vi "EnableDisableBankB - Right Click.vi"(8 "error in (no error)":errorcluster, 11 "Node Ptr":u64 format="%.0x") -> (0 "error out":errorcluster)   [LabVIEW 2015, in "DCM System Explorer.lvlib"]
uses:
  DCM System Explorer.lvlib
  System.Windows.Forms
  Shared/DCM Constants and GUIDs.vi
  Shared/DCM Properties.vi
  <vilib>/NI Veristand/Custom Device API/Set Item Property (Boolean).vi
  <vilib>/NI VeriStand/Custom Device API/Custom Device API.lvlib
  DCM Shared.lvlib
  <vilib>/NI Veristand/Custom Device Tools/Custom Device Utility Library/Custom Device Utility Library.lvlib
panel:
  in  "Tag":string
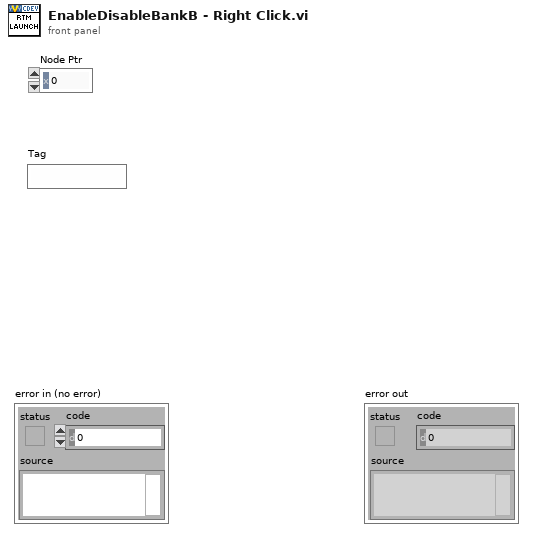
[diagram p1: front panel]
types:
  T1 = typedef "Custom Device API.lvlib/Custom Device Item Ref.ctl" = u64
  T2 = typedef "DCM - RT - DI.lvlib/Command.ctl" = cluster{"Mode":T3, "Digital Input":T4, "Default Phase Index":u8, "Frequency [Hz]":sgl, "Duration [s]":sgl, "Sweep [s]":sgl, "Injections":u16, "Command Sequence":T5[], "TDC Offset [CAD]":sgl, "Window Start [DBTDC]":sgl, "Window End [DBTDC]":sgl, "Angles":T6[], "Skip Fire":bool, "Skip Fire Index":u8}
  T3 = typedef "DCM - FPGA - DI.lvlib/Mode.ctl" = enum8{"Off", "Direct", "Calibration", "Triggered Multi-Pulse", "Engine Position Tracking"}
  T4 = typedef "DCM - FPGA.lvlib/Digital Channel.ctl" = enum8{"Unused", "Diff IO 1", "Diff IO 2", "Diff IO 3", "Diff IO 4", "Diff IO 5", "Diff IO 6", "Diff IO 7", "Diff IO 8", "Aux 1", "Aux 2", "Aux 3", "Aux 4", "Aux 5", "Aux 6", "Aux 7", "Aux 8", "User OS"}
  T5 = typedef "DCM - RT - DI.lvlib/Command Sequence.ctl" = cluster{"Duration [s]":sgl, "CmdLevel":bool, "Run":bool, "Phase Index":u8}
  T6 = typedef "DCM - RT - DI.lvlib/Angle Control.ctl" = cluster{"Enable":bool, "Location [DBTDC]":sgl, "Duration [s]":sgl, "Phase Index":u8}
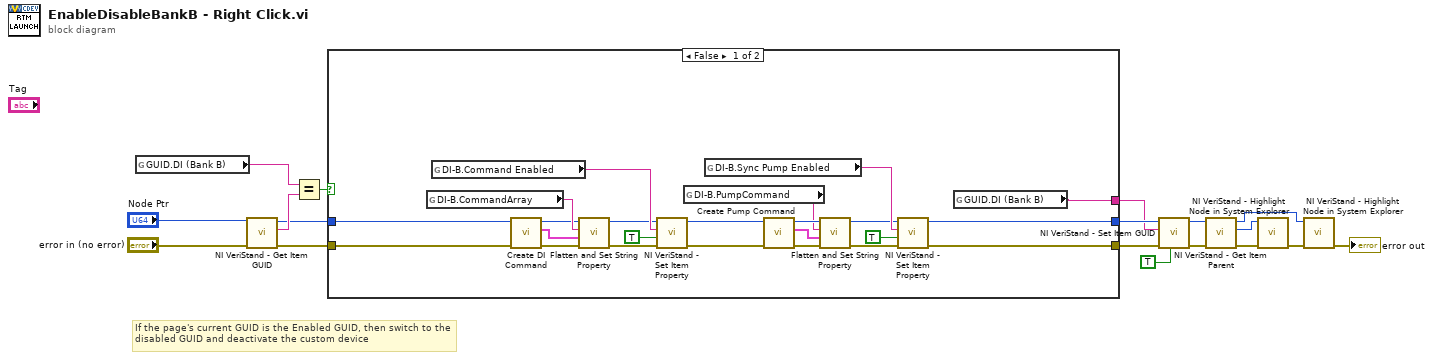
[diagram p0: block diagram]
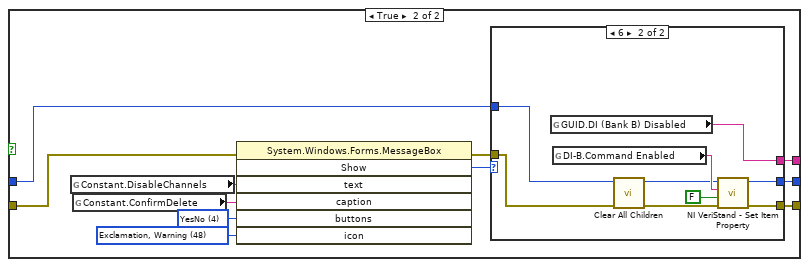
[diagram p2: hidden frame]
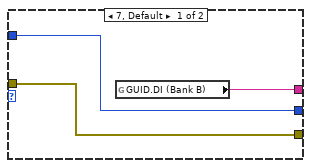
[diagram p3: hidden frame]
diagram:
  # "If the page's current GUID is the Enabled GUID, then switch to the disabled GUID and deactivate the custom device"
  n1 = global read "DCM Constants and GUIDs.vi" "GUID.DI (Bank B)"() -> (w15:string)
  n2 = call <vilib>:"NI VeriStand - Get Item GUID.vi"("error in (no error)"="error in (no error)", "Item Ref in"="Node Ptr") -> ("error out"=w13:errorcluster, "GUID"=w18:string, "Item Ref out"=w14:T1)  [unwired: 7 in]
  n3 = Equal?(x=w15, y=w18) -> (x = y?=w1:bool)
  n4 = case shown="False" w1 {
    tunnel: w13 -> [w41 w48]
    tunnel: [w20 w45] -> w10
    tunnel: w14 -> [w38 w44]
    tunnel: [w19 w42] -> w11
    tunnel: [w31 w43] -> w9
    frame False {
      n5 = global read "DCM Properties.vi" "DI-B.CommandArray"() -> (w37:string)
      n6 = global read "DCM Properties.vi" "DI-B.Command Enabled"() -> (w40:string)
      n7 = call "Create DI Command.vi"("error in (no error)"=w41, "Section Ptr"=w38) -> ("error out"=w35:errorcluster, "Command"=w32:T2[], "Parent Ref out"=w36:T1)  [unwired: 6 in, 1 out]
      n8 = call "Flatten and Set String Property.vi"("error in (no error)"=w35, "Value"=w32, "Property Name"=w37, "Section Ref in"=w36) -> ("error out"=w34:errorcluster, "Section Ref out"=w33:T1)  [unwired: 6 in]
      n9 = call-poly <vilib>:"NI VeriStand - Set Item Property.vi"("error in (no error)"=w34, "Value"=TRUE, "Property Name"=w40, "Item Ref in"=w33) -> ("error out"=w21:errorcluster, "Item Ref out"=w22:T1)  [unwired: 5 in, 1 out]
      n10 = global read "DCM Properties.vi" "DI-B.PumpCommand"() -> (w24:string)
      n11 = global read "DCM Properties.vi" "DI-B.Sync Pump Enabled"() -> (w30:string)
      n12 = call "Create Pump Command.vi"("error in (no error)"=w21, "Section Ptr"=w22) -> ("error out"=w27:errorcluster, "Pump Command"=w23:T2, "Parent Ref out"=w28:T1)  [unwired: 7 in]
      n13 = call "Flatten and Set String Property.vi"("error in (no error)"=w27, "Value"=w23, "Property Name"=w24, "Section Ref in"=w28) -> ("error out"=w25:errorcluster, "Section Ref out"=w26:T1)  [unwired: 6 in]
      n14 = call-poly <vilib>:"NI VeriStand - Set Item Property.vi"("error in (no error)"=w25, "Value"=TRUE, "Property Name"=w30, "Item Ref in"=w26) -> ("error out"=w20:errorcluster, "Item Ref out"=w19:T1)  [unwired: 5 in, 1 out]
      n15 = global read "DCM Constants and GUIDs.vi" "GUID.DI (Bank B)"() -> (w31:string)
    }
    frame True {
      w49 = 4 items=["OK", "OKCancel", "AbortRetryIgnore", "YesNoCancel", "YesNo", "RetryCancel"] ("buttons")
      w50 = 48 items=["None"=0, "Hand, Error, Stop"=16, "Question"=32, "Exclamation, Warning"=48, "Asterisk, Information"=64] ("icon")
      n16 = global read "DCM Constants and GUIDs.vi" "Constant.DisableChannels"() -> (w51:string)
      n17 = global read "DCM Constants and GUIDs.vi" "Constant.ConfirmDelete"() -> (w52:string)
      n18 = invoke class="System.Windows.Forms.MessageBox" method="Show"(error in=w48, "text"=w51, "caption"=w52, "buttons"=w49, "icon"=w50) -> (error out=w46:errorcluster, "Show"=w47:i32)  [unwired: 2 in, 5 out]
      n19 = case shown="6" w47 {
        tunnel: w46 -> [w55 w64]
        tunnel: [w55 w61] -> w45
        tunnel: w44 -> [w53 w63]
        tunnel: [w54 w57] -> w43
        tunnel: [w53 w56] -> w42
        frame 7, Default {
          n20 = global read "DCM Constants and GUIDs.vi" "GUID.DI (Bank B)"() -> (w54:string)
        }
        frame 6 {
          n21 = global read "DCM Constants and GUIDs.vi" "GUID.DI (Bank B) Disabled"() -> (w57:string)
          n22 = global read "DCM Properties.vi" "DI-B.Command Enabled"() -> (w60:string)
          n23 = call "Clear All Children.vi"("error in (no error)"=w64, "Item Ref in"=w63) -> ("error out"=w62:errorcluster, "Item Ref out"=w58:T1)  [unwired: 8 in]
          n24 = call-poly <vilib>:"NI VeriStand - Set Item Property.vi"("error in (no error)"=w62, "Value"=FALSE, "Property Name"=w60, "Item Ref in"=w58) -> ("error out"=w61:errorcluster, "Item Ref out"=w56:T1)  [unwired: 5 in, 1 out]
        }
      }
    }
  }
  n25 = call <vilib>:"NI VeriStand - Set Item GUID.vi"("Refresh System Explorer Tree? (F)"=TRUE, "error in (no error)"=w10, "GUID"=w9, "Item Ref in"=w11) -> ("error out"=w6:errorcluster, "Item Ref out"=w5:T1)  [unwired: 6 in]
  n26 = call <vilib>:"NI VeriStand - Get Item Parent.vi"("error in (no error)"=w6, "Item Ref in"=w5) -> ("error out"=w7:errorcluster, "Parent Ref"=w8:T1, "Item Ref out"=w2:T1)  [unwired: 6 in, 1 out]
  n27 = call <vilib>:"NI VeriStand - Highlight Node in System Explorer.vi"("error in (no error)"=w7, "Item Ref in"=w8) -> ("error out"=w4:errorcluster)  [unwired: 8 in, 1 out]
  n28 = call <vilib>:"NI VeriStand - Highlight Node in System Explorer.vi"("error in (no error)"=w4, "Item Ref in"=w2) -> ("error out"=→"error out":errorcluster)  [unwired: 8 in, 1 out]
